vi "Set Continuity Enabled.vi"(8 "error in (no error)":errorcluster, 10 "Continuity Enabled":bool, 11 "VISA resource name":refnum<visa-resource-name>) -> (0 "error out":errorcluster, 3 "VISA resource name out":refnum<visa-resource-name>)   [LabVIEW 2020, in "Associated Research 78XX Series.lvlib"]
uses:
  <instrlib>/Associated Research 78XX Series/Associated Research 78XX Series.lvlib
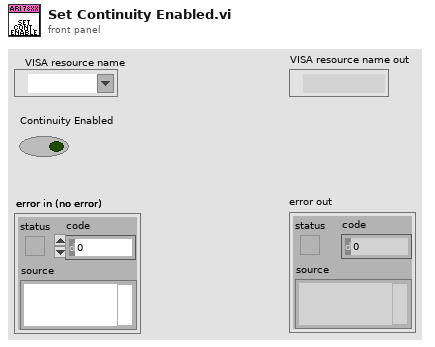
[diagram p1: front panel]
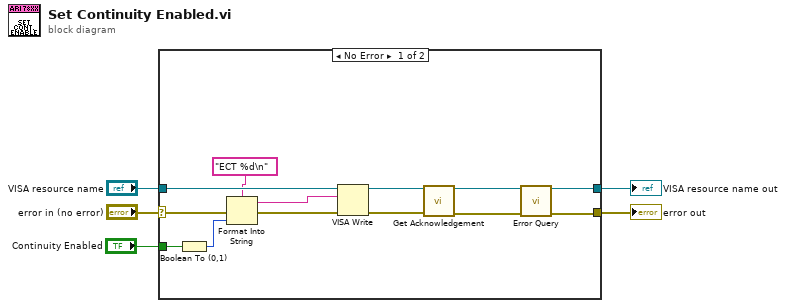
[diagram p0: block diagram]
diagram:
  n1 = case shown="No Error" "error in (no error)" {
    selector: "error in (no error)" -> [w16 w20]
    tunnel: [w15 w20] -> w4
    tunnel: [w17 w19] -> w2
    tunnel: "VISA resource name" -> [w18 w19]
    tunnel: "Continuity Enabled" -> [w7 _]
    frame No Error {
      n2 = Boolean To (0,1)(Boolean=w7) -> (0, 1=w6:i16)
      n3 = Format Into String(format string="ECT %d\n" ("\"False\" Command"), error in=w16, w6) -> (resulting string=w10:string, error out=w13:errorcluster)  [unwired: 1 in]
      n4 = VISA Write(VISA resource name=w18, write buffer=w10, error in (no error)=w13) -> (VISA resource name out=w9:refnum<visa-resource-name>, error out=w8:errorcluster)  [unwired: 1 out]
      n5 = call <instrlib>:"Get Acknowledgement.vi"("VISA resource name"=w9, "error in (no error)"=w8) -> ("VISA resource name out"=w12:refnum<visa-resource-name>, "error out"=w11:errorcluster)  [unwired: 12 in]
      n6 = call <instrlib>:"Error Query.vi"("VISA resource name"=w12, "error in (no error)"=w11) -> ("VISA resource name out"=w17:refnum<visa-resource-name>, "error out"=w15:errorcluster)  [unwired: 10 in, 2 out]
    }
    frame Error {
    }
  }
  "error out" <- w4
  "VISA resource name out" <- w2
